vi "UpdateTextFile_timestamp_string.vi"(0 "string":string, 2 "file path":path) -> ()   [LabVIEW 2018]
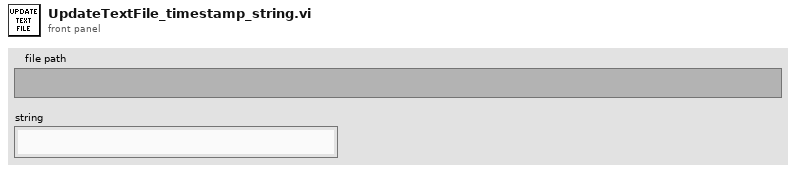
[diagram p1: front panel]
types:
  T1 = enum16{"open", "open or create", "create or replace", "create", "open (read only)"}
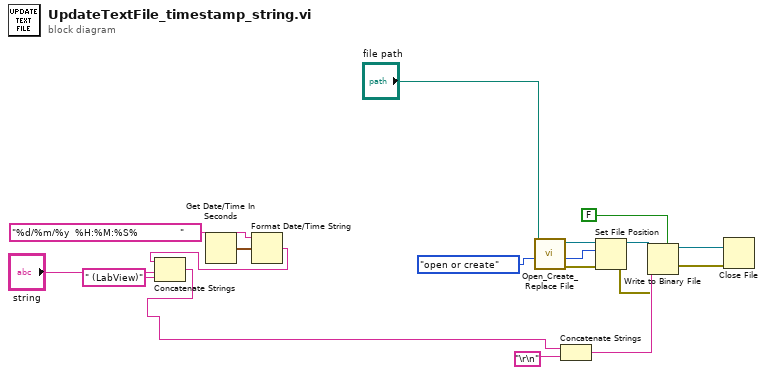
[diagram p0: block diagram]
diagram:
  n1 = Get Date/Time In Seconds() -> (seconds since 1Jan1904=w7:timestamp)
  n2 = Format Date/Time String(time format string (%c)="%d/%m/%y  %H:%M:%S%              ", seconds (now)=w7) -> (date/time string=w6:string)  [unwired: 1 in]
  n3 = Concatenate Strings(w6, "string", " (LabView)" ("string")) -> (w4:string)
  n4 = call <vilib>:"Open_Create_Replace File.vi"("function (open:0)"=T1."open or create", "file path"="file path") -> ("error out"=w17:errorcluster, "file size (bytes)"=w15:i32, "refnum"=w16:refnum<file>)  [unwired: 6 in, 1 out]
  n5 = Concatenate Strings(w4, "\r\n") -> (w11:string)
  n6 = Set File Position(offset (in bytes) (0)=w15, refnum=w16, error in=w17) -> (refnum out=w10:refnum<file>, error out=w9:errorcluster)  [unwired: 1 in]
  n7 = Write to Binary File(file (use dialog)=w10, data=w11, error in=w9, 5:FALSE ("prepend array or string size? (T)")) -> (refnum out=w13:refnum<file>, error out=w14:errorcluster)  [unwired: 2 in, 1 out]
  n8 = Close File(refnum=w13, error in=w14) -> ()  [unwired: 2 out]
